vi "Convert.vi"(11 "Data":u8[](array[numeric])) -> (3 "Value":dbl)   [LabVIEW 2024]
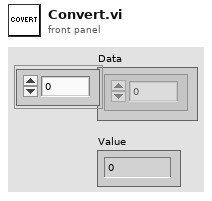
[diagram p1: front panel]
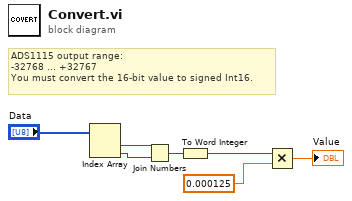
[diagram p0: block diagram]
diagram:
  # "ADS1115 output range:\n-32768 ... +32767\nYou must convert the 16-bit value to signed Int16."
  n1 = Index Array(array="Data") -> (element #1=w5:u8, element #2=w6:u8)  [unwired: 2 in]
  n2 = Join Numbers(hi=w5, lo=w6) -> ((hi.lo)=w7:u16)
  n3 = To Word Integer(number=w7) -> (16bit integer=w1:i16)
  n4 = Multiply(x=w1, y=0.000125) -> (x*y=→"Value":dbl)
